vi "Clear Attributes Memory.vi"(8 "error in (no error)":errorcluster, 11 "UIConfiguration in":refnum<class "UIConfiguration.lvclass">) -> (0 "error out":errorcluster, 3 "UIConfiguration out":refnum<class "UIConfiguration.lvclass">)   [LabVIEW 2015, in "UIConfiguration.lvclass"]
uses:
  UIConfiguration.lvclass
  UIConfiguration.lvclass/UIConfiguration.ctl
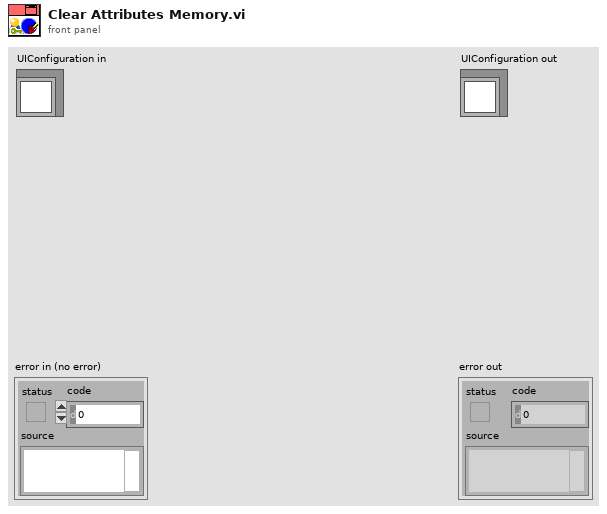
[diagram p1: front panel]
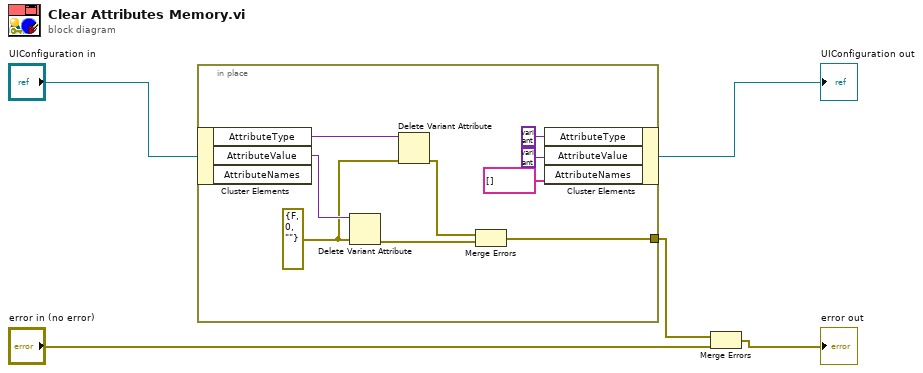
[diagram p0: block diagram]
diagram:
  n1 = in-place {
    in-place-border: [w6] -> w2
    w9 = errorcluster {"status"=FALSE, "code"=0, "source"=""} ("error constant")
    n2 = in-place-cluster #1("UIConfiguration in") -> ("AttributeType"=w11:variant, "AttributeValue"=w10:variant)  [unwired: 1 out]
    n3 = Delete Variant Attribute(4:w9, 7:w10) -> (0:w7:errorcluster)  [unwired: 1 in, 2 out]
    n4 = Delete Variant Attribute(4:w9, 7:w11) -> (0:w8:errorcluster)  [unwired: 1 in, 2 out]
    n5 = Merge Errors(w8, w7) -> (w6:errorcluster)
    n6 = in-place-cluster #1("AttributeType"=variant, "AttributeValue"=variant, "AttributeNames"=string[] []) -> (→"UIConfiguration out":refnum<class "UIConfiguration.lvclass">)
  }
  n7 = Merge Errors(w2, "error in (no error)") -> (→"error out":errorcluster)
